vi "Hood to Angle.vi"(11 "Hood Angle":dbl) -> (3 "Encoder":dbl)   [LabVIEW 2019]
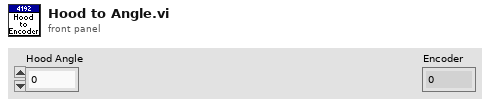
[diagram p1: front panel]
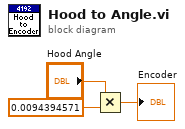
[diagram p0: block diagram]
diagram:
  n1 = Multiply(x="Hood Angle", y=0.0094394571) -> (x*y=→"Encoder":dbl)
